vi "Parse Xeryon STAT.vi"() -> ()   [LabVIEW 2019]
panel:
  out "STAT":string[][](table)
  in  "STAT Word":string
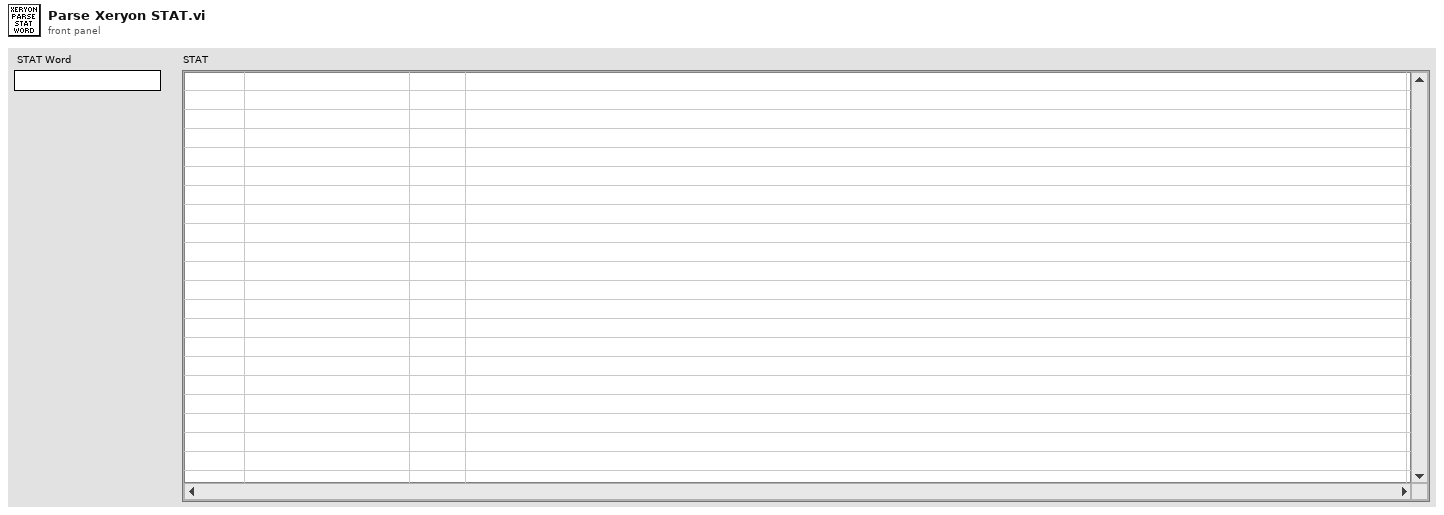
[diagram p1: front panel]
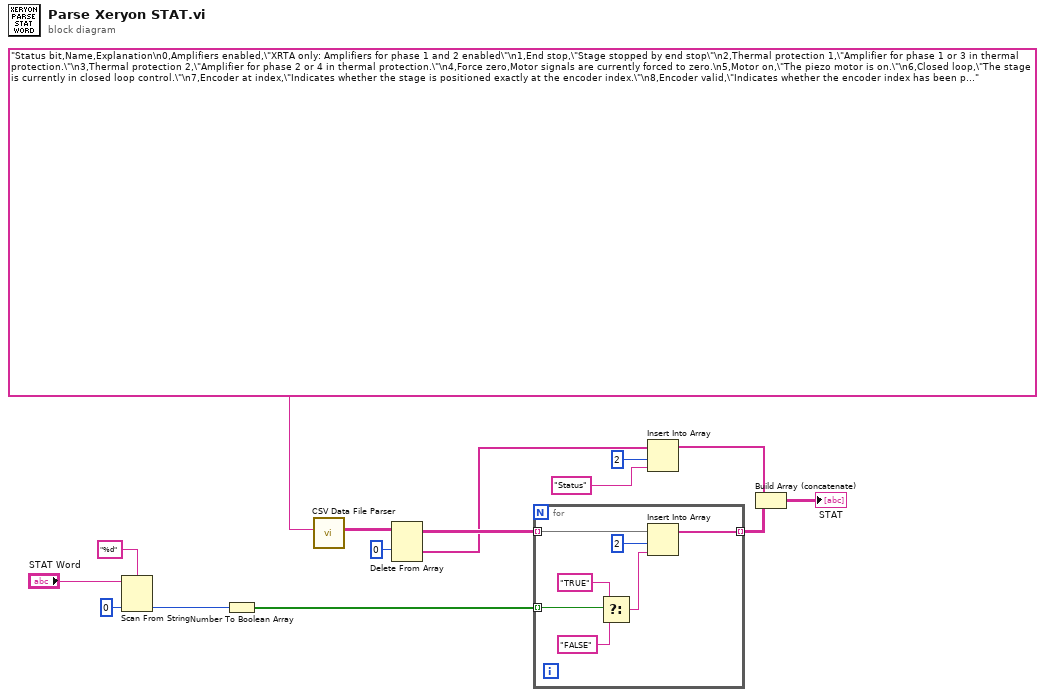
[diagram p0: block diagram]
diagram:
  n1 = Scan From String(format string="%d", input string="STAT Word", default 1=0 ("default value 1")) -> (output 1=w12:i32)  [unwired: 2 in, 3 out]
  n2 = Number To Boolean Array(number=w12) -> (Boolean array=w7:bool[])
  n3 = call "CSV Data File Parser.vi"("CSV String"="Status bit,Name,Explanation\n0,Amplifiers enabled,\"XRTA only: Amplifiers for phase 1 and 2 enabled\"\n1,End stop,\"Stage stopped by end stop\"\n2,Thermal protection 1,\"Amplifier for phase 1 or 3 in thermal protection.\"\n3,Thermal protection 2,\"Amplifier for phase 2 or 4 in thermal protection.\"\n4,Force zero,Motor signals are currently forced to zero.\n5,Motor on,\"The piezo motor is on.\"\n6,Closed loop,\"The stage is currently in closed loop control.\"\n7,Encoder at index,\"Indicates whether the stage is positioned exactly at the encoder index.\"\n8,Encoder valid,\"Indicates whether the encoder index has been passed and therefore the encoder value reflects the absolute position, not the relative position with respect to the startup position.\"\n9,Searching index,\"Indicates whether the stage is currently searching the index position.\"\n10,Position reached,\"Indicates whether the target position is reached (within tolerance limits).\"\n11,Error compensation,\"Error compensation is on.\"\n12,Encoder error,\"Indicates an error produced by the encoder.\"\n13,Scanning,\"Indicates whether the stage is in a scanning mode.\"\n14,Left end stop,\"Indicates that the left end stop is passed.\"\n15,Right end stop,\"Indicates that the right end stop is passed.\"\n16,Error limit,\"Indicates that the position error has reached the limit set by ELIM. This can indicate a collision or mechanical limit (end of stroke).\"\n17,Searching optimal frequency,\"The driver is searching for the optimal excitation frequency of the piezo motor.\"\n18,Safety timeout triggered,\"If this is set to '1', then the safety timeout was triggered. See the explanation of the command 'TOU2' several pages back.\"\n19,EtherCAT acknowledge,\"only used when control via EtherCAT\"\n20,Emergency stop,\"not used\"\n21,Position fail,\"If this is set to '1', then the safety timeout TOU3 was triggered.\"") -> ("2-D Array"=w10:string[][])  [unwired: 8 in, 2 out]
  n4 = Delete From Array(array=w10, index (row)=0) -> (deleted portion=w6:string[], array with subset deleted=w8:string[][])  [unwired: 2 in]
  n5 = for {
    tunnel: w8 -> [w19] mode=indexing
    tunnel: w7 -> [w22] mode=indexing
    tunnel: [w16] -> w2 mode=indexing
    n6 = Select(t="TRUE", s=w22, f="FALSE") -> (s? t:f=w18:string)
    n7 = Insert Into Array(array=w19, index=2, new element=w18) -> (w16:string[])
  }
  n8 = Insert Into Array(array=w6, index=2, new element="Status" ("new element/subarray")) -> (w3:string[])
  n9 = Build Array (concatenate)(w3, w2) -> (→"STAT":string[][])
